vi "demo.vi"() -> ()   [LabVIEW 2019]
uses:
  <vilib>/Platform/storage/lvStorage.llb/_openFunction.ctl
  <vilib>/Platform/storage/lvStorage.llb/_openStorageWithRootAutoDetect.vi
  <vilib>/Platform/storage/lvStorage.llb/xStorage/xStorageSupp/ErrorOut.vi
  <vilib>/Platform/storage/lvStorage.llb/_queryPropPoly.vi
  <vilib>/Platform/storage/lvStorage.llb/_queryPropString.vi
  <vilib>/Platform/storage/lvStorage.llb/_queryGenericObjects.vi
  <vilib>/Platform/storage/lvStorage.llb/_loadAllDouble.vi
  <vilib>/Platform/storage/lvStorage.llb/_loadAllDdt.vi
  <vilib>/Platform/storage/Storage.llb/Get Object Info.vi
  <vilib>/Platform/storage/Storage.llb/__closeStorageFromObject.vi
  <vilib>/Instr/_visa.llb/VISA Configure Serial Port (Instr).vi
  <vilib>/Utility/file.llb/Write Delimited Spreadsheet (I64).vi
  <vilib>/Platform/storage/lvStorage.llb/xStorage/Open Data Storage/Open Data Storage.xnode
  <vilib>/Platform/storage/lvStorage.llb/xStorage/Read Data/Read Data.xnode
  <vilib>/Platform/storage/lvStorage.llb/xStorage/Close Data Storage/Close Data Storage.xnode
  phlib64.dll
panel:
  in  "If NLOS":bool
  out "Numeric":dbl
  out "String":string
  out "Index":dbl
  out "Histogram":u32[](graph)
  out "DLL Version (must be 3.0)":string caption="DLL Version"
  out "Calibration Status":string
  out "Initialization Status":string
  # "1: NLOS\n0: LOS"
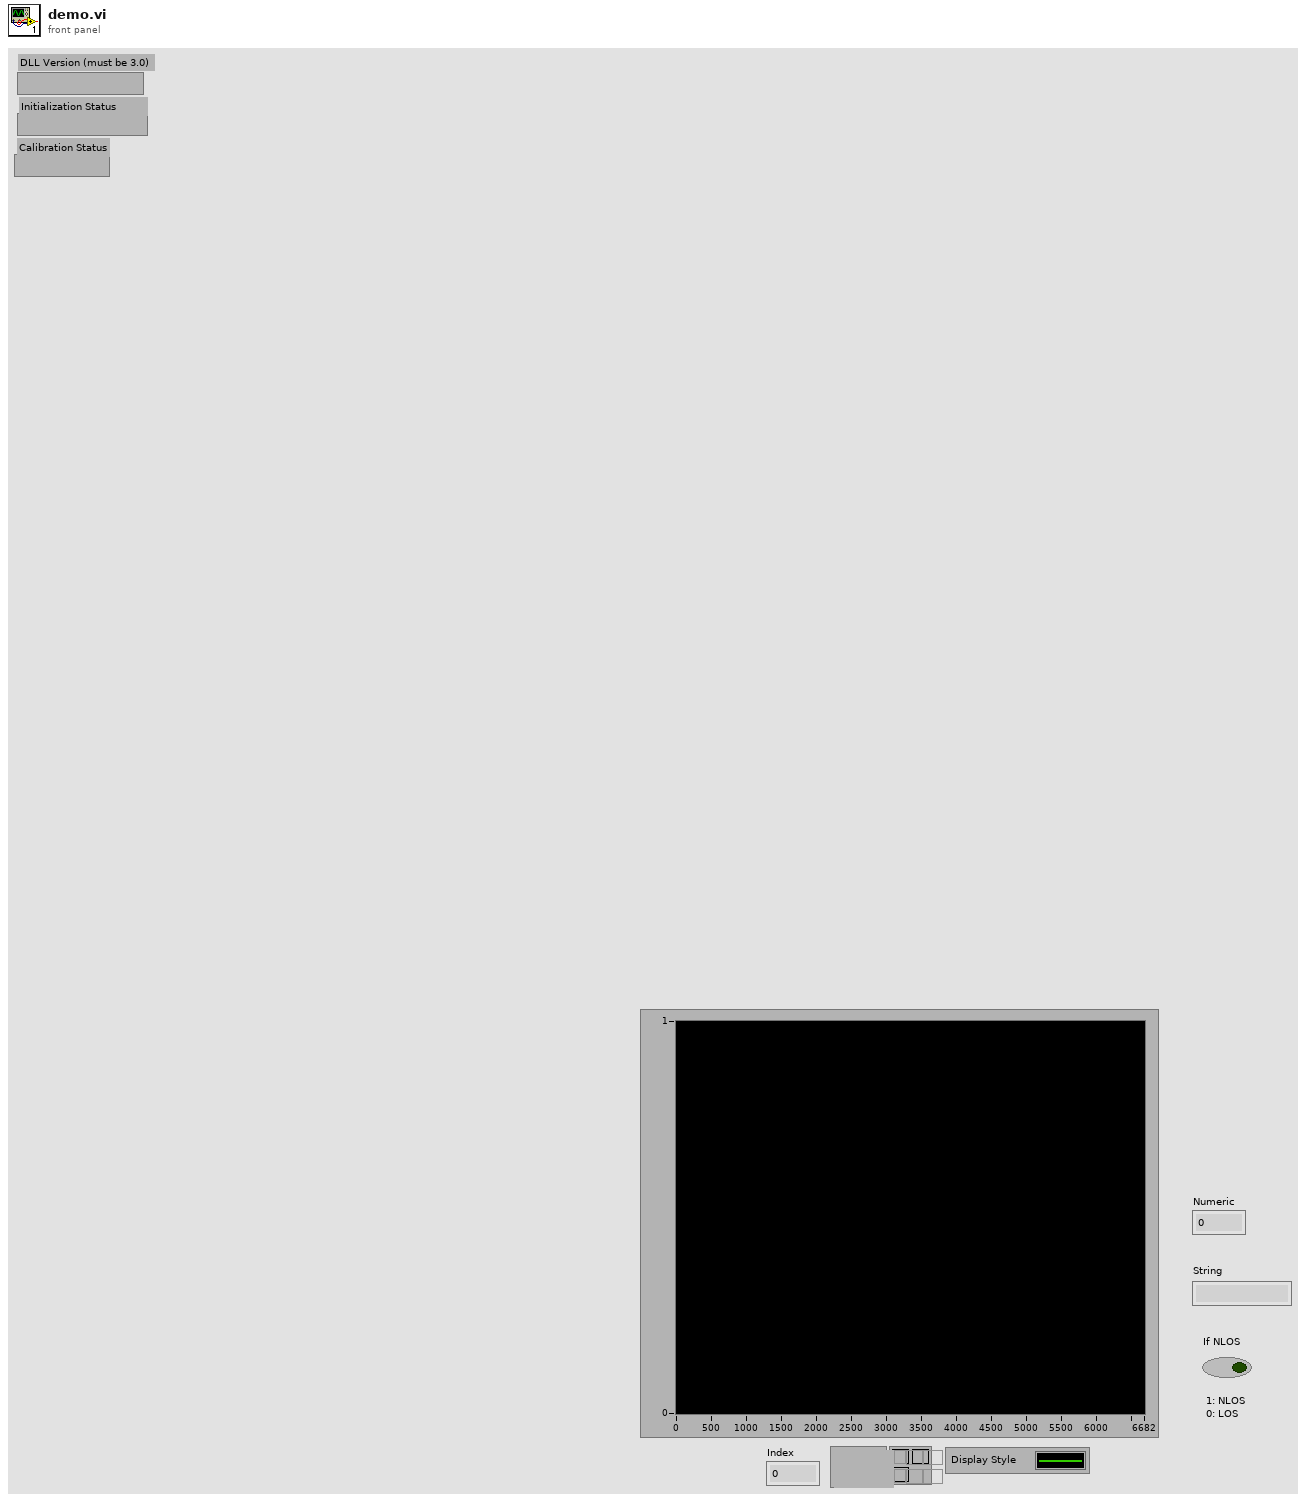
[diagram p1: front panel]
types:
  T1 = enum16{"UPDATE", "READ", "QUERY", "CREATE CHILD", "CREATE", "CONNECT", "DISCONNECT"}
  T2 = typedef "_openFunction.ctl" = enum16{"open", "open or create", "create or replace", "create", "open (read only)"}
  T3 = enum16{"open", "replace", "create", "open or create", "replace or create", "replace or create with confirmation"}
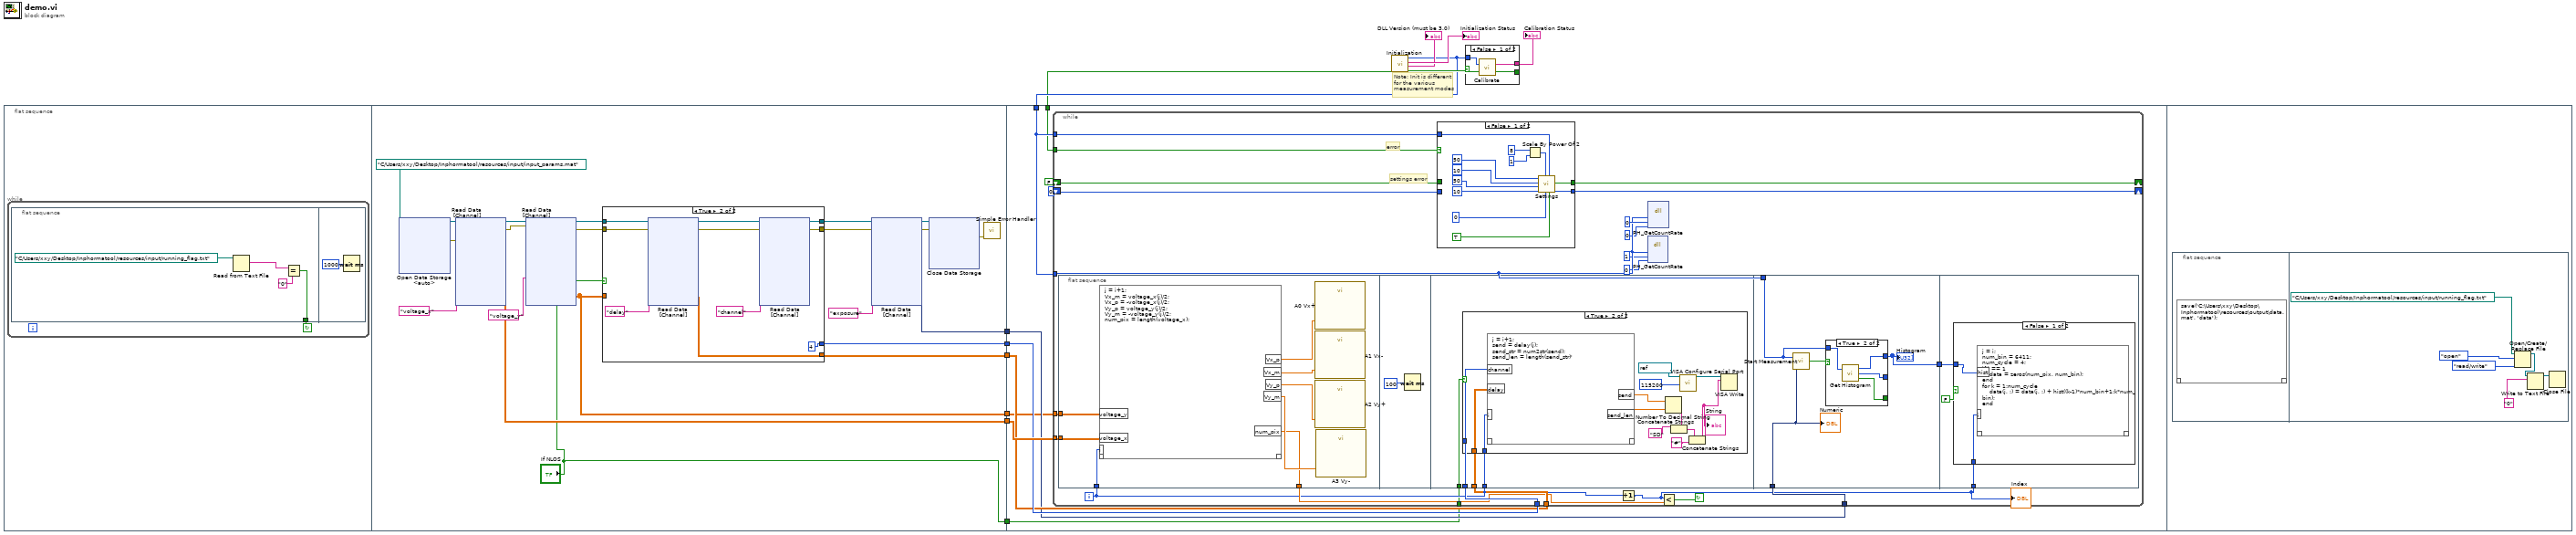
[diagram p0: block diagram]
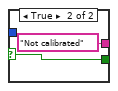
[diagram p2: hidden frame]
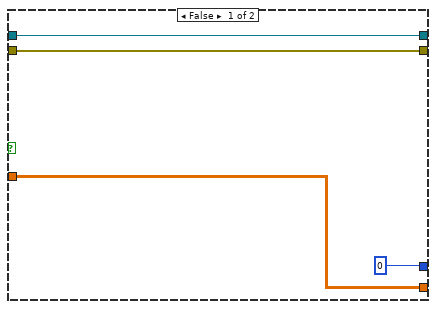
[diagram p3: hidden frame]
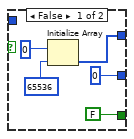
[diagram p5: hidden frame]
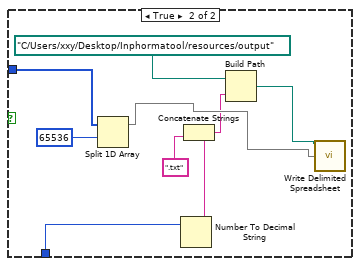
[diagram p6: hidden frame]
diagram:
  # "Note: Init is different \nfor the various\nmeasurement modes"
  n1 = flat-sequence {
    tunnel: [w36] -> w12
    tunnel: [w35] -> w11
    tunnel: [w34] -> w10
    tunnel: [w30] -> w9
    tunnel: [w21] -> w2
    tunnel: ["If NLOS"] -> w1
    tunnel: w4 -> [w171]
    tunnel: w3 -> [w170]
    tunnel: w9 -> [w164]
    tunnel: w10 -> [w166]
    tunnel: w11 -> [w165]
    tunnel: w12 -> [w167]
    tunnel: w2 -> [w163]
    tunnel: w1 -> [w162]
    frame #0 {
      n2 = while {
        stop <- w13 continue-if-true
        n3 = flat-sequence {
          tunnel: [w15] -> w13
          frame #0 {
            n4 = Read from Text File(file (use dialog)=path "C:/Users/xxy/Desktop/Inphormatool/resources/input/running_flag.txt") -> (text=w14:string)  [unwired: 3 in, 3 out]
            n5 = Equal?(x=w14, y="0") -> (x = y?=w15:bool)
          }
          frame #1 {
            n6 = Wait (ms)(milliseconds to wait=1000) -> ()  [unwired: 1 out]
          }
        }
      }
    }
    frame #1 {
      n7 = xnode "Open Data Storage\n<auto>"("file path"=path "C:/Users/xxy/Desktop/Inphormatool/resources/input/input_params.mat") -> ("storage refnum (file)"=w39:refnum<k20>, "error out"=w38:errorcluster)  [unwired: 4 in, 1 out]
      n8 = xnode "Read Data\n[Channel]"("Name"="voltage_x", "storage refnum (file)"=w39, "error in"=w38) -> ("Signal"=w36:dbl[][], "storage refnum (file) out"=w26:refnum<k20>, "error out"=w25:errorcluster)  [unwired: 3 in, 1 out]
      n9 = xnode "Read Data\n[Channel]"("Name"="voltage_y", "storage refnum (file)"=w26, "error in"=w25) -> ("Signal"=w21:dbl[][], "storage refnum (file) out"=w24:refnum<k20>, "error out"=w23:errorcluster)  [unwired: 3 in, 1 out]
      n10 = case shown="True" "If NLOS" {
        tunnel: w24 -> [w61 w71]
        tunnel: w23 -> [w60 w70]
        tunnel: [w58 w65] -> w35
        tunnel: [0 4] -> w34
        tunnel: [w61 w64] -> w32
        tunnel: [w60 w63] -> w31
        tunnel: w21 -> [w58 _]
        frame False {
        }
        frame True {
          n11 = xnode "Read Data\n[Channel]"("Name"="delay", "storage refnum (file)"=w71, "error in"=w70) -> ("Signal"=w65:dbl[][], "storage refnum (file) out"=w67:refnum<k20>, "error out"=w66:errorcluster)  [unwired: 3 in, 1 out]
          n12 = xnode "Read Data\n[Channel]"("Name"="channel", "storage refnum (file)"=w67, "error in"=w66) -> ("storage refnum (file) out"=w64:refnum<k20>, "error out"=w63:errorcluster)  [unwired: 3 in, 2 out]
        }
      }
      n13 = xnode "Read Data\n[Channel]"("Name"="exposure", "storage refnum (file)"=w32, "error in"=w31) -> ("Signal"=w30:dynamicdata, "storage refnum (file) out"=w28:refnum<k20>, "error out"=w27:errorcluster)  [unwired: 3 in, 1 out]
      n14 = xnode "Close Data Storage\n"("storage refnum (file)"=w28, "error in (no error)"=w27) -> ("error out"=w29:errorcluster)  [unwired: 1 out]
      n15 = call <vilib>:"Simple Error Handler.vi"("error in (no error)"=w29) -> ()  [unwired: 4 in, 5 out]
    }
    frame #2 {
      n16 = while {
        shift-right: [w189] -> _
        shift-left: FALSE -> [w190]
        shift-right: [w193] -> _
        shift-left: 0 -> [w192]
        tunnel: w170 -> [w191]
        tunnel: w171 -> [w188]
        tunnel: w171 -> [w186]
        tunnel: w167 -> [w182]
        tunnel: w166 -> [w181]
        tunnel: w165 -> [w178]
        tunnel: w164 -> [w180]
        tunnel: w163 -> [w177]
        tunnel: w162 -> [w172]
        i -> [w174]
        stop <- w175 continue-if-true
        # "settings error"
        # "error"
        n17 = flat-sequence {
          tunnel: w174 -> [w201]
          tunnel: w182 -> [w196]
          tunnel: w177 -> [w195]
          tunnel: [w194] -> w176
          tunnel: w181 -> [w205]
          tunnel: w178 -> [w206]
          tunnel: w174 -> [w204]
          tunnel: w172 -> [w203]
          tunnel: w186 -> [w223]
          tunnel: w180 -> [w220]
          tunnel: [w221] -> w179
          tunnel: w179 -> [w235]
          tunnel: w173 -> [w234]
          frame #0 {
            n18 = script code="j = i+1;\nVx_m = voltage_x(j)/2;\nVx_p = -voltage_x(j)/2;\nVy_p = voltage_y(j)/2;\nVy_m = -voltage_y(j)/2;\nnum_pix = length(voltage_x);"("voltage_x"=w196, "i"=w201, "voltage_y"=w195) -> ("Vx_p"=w200:dbl, "Vx_m"=w199:dbl, "Vy_p"=w198:dbl, "Vy_m"=w197:dbl, "num_pix"=w194:dbl)  [unwired: 1 in, 1 out]
            n19 = call "A0 Vx+"("data"=w200) -> ()  [unwired: 17 in, 2 out]
            n20 = call "A1 Vx-"("data"=w199) -> ()  [unwired: 17 in, 2 out]
            n21 = call "A2 Vy+"("data"=w198) -> ()  [unwired: 17 in, 2 out]
            n22 = call "A3 Vy-"("data"=w197) -> ()  [unwired: 17 in, 2 out]
          }
          frame #1 {
            n23 = Wait (ms)(milliseconds to wait=100) -> ()  [unwired: 1 out]
          }
          frame #2 {
            n24 = case shown="True" w203 {
              tunnel: w206 -> [_ w215]
              tunnel: w205 -> [_ w217]
              tunnel: w204 -> [_ w216]
              frame False {
              }
              frame True {
                n25 = script code="j = i+1;\nsend = delay(j);\nsend_str = num2str(send);\nsend_len = length(send_str)'"("channel"=w217, "delay"=w215, "i"=w216) -> ("send"=w213:dbl, "send_len"=w207:dbl)  [unwired: 1 in, 1 out]
                n26 = Number To Decimal String(number=w213, width (-)=w207) -> (decimal integer string=w211:string)
                n27 = Concatenate Strings("SD", w211) -> (w210:string)
                n28 = call-poly "VISA Configure Serial Port"("VISA resource name"=refnum<visa-resource-name> "COM8", "baud rate (9600)"=u32 115200) -> ("VISA resource name out"=w218:refnum<visa-resource-name>)  [unwired: 12 in, 1 out]
                n29 = Concatenate Strings(w210, "#") -> (w209:string)
                "String" <- w209
                n30 = VISA Write(VISA resource name=w218, write buffer=w209) -> ()  [unwired: 1 in, 3 out]
              }
            }
          }
          frame #3 {
            n31 = call "Start Measurement.vi"("Acquisition time"=w220, "DeviceIndex"=w223) -> ("DataValid"=w222:bool)
            n32 = case shown="True" w222 {
              tunnel: [w227 w232] -> w221
              tunnel: [FALSE w230] -> _
              tunnel: [u32 0 w231] -> _
              tunnel: w223 -> [_ w229]
              frame False {
                n33 = Initialize Array "Initialize Array"(u32 0, 65536) -> (w227:u32[])
              }
              frame True {
                n34 = call "Get Histogram.vi"("DeviceIndex"=w229) -> ("Histogram"=w232:u32[], "IntegralCount"=w231:i32, "Overflow"=w230:bool)  [unwired: 1 in]
              }
            }
            "Histogram" <- w221
            "Numeric" <- w220
          }
          frame #4 {
            n35 = case shown="False" FALSE {
              tunnel: w235 -> [w237 w241]
              tunnel: w234 -> [w236 w239]
              frame False {
                n36 = script code="j = i;\nnum_bin = 6411;\nnum_cycle = 4;\nif j == 1\n    data = zeros(num_pix, num_bin);\nend\nfor k = 1:num_cycle\n    data(j, :) = data(j, :) + hist((k-1)*num_bin+1:k*num_bin);\nend"("hist"=w237, "i"=w236) -> ()  [unwired: 1 in, 1 out]
              }
              frame True {
                n37 = Split 1D Array(array=w241, index=65536) -> (first subarray=w246:u32[])  [unwired: 1 out]
                n38 = Number To Decimal String(number=w239) -> (decimal integer string=w240:string)  [unwired: 1 in]
                n39 = Concatenate Strings(w240, ".txt") -> (w244:string)
                n40 = Build Path(base path=path "C:/Users/xxy/Desktop/Inphormatool/resources/output", name or relative path=w244) -> (appended path=w245:path)
                n41 = call-poly <vilib>:"Write Delimited Spreadsheet.vi"("file path (dialog if empty)"=w245, "1D data"=w246) -> ()  [unwired: 12 in, 2 out]
              }
            }
          }
        }
        n42 = case shown="False" w191 {
          tunnel: [w258 w260] -> w189
          tunnel: w190 -> [_ w260]
          tunnel: [w257 w259] -> w193
          tunnel: w192 -> [_ w259]
          tunnel: w188 -> [w254 _]
          frame False {
            n43 = Scale By Power Of 2(n=8, x=1) -> (x*2^n=w255:i32)
            n44 = call "Settings.vi"("StopOnOverflow"=TRUE, "DeviceIndex"=w254, "Range No."=0, "SyncDiv"=w255, "CFD1 zero X"=10, "CFD1 level"=50, "CFD0 zero X"=10, "CFD0 level"=50) -> ("Resolution"=w257:i32, "Error"=w258:bool)  [unwired: 2 in]
          }
          frame True {
          }
        }
        n45 = Increment(x=w174) -> (x+1=w173:i32)
        "Index" <- w173
        n46 = dll-call lib="PHLib64.dll" fn="PH_GetCountRate"("devidx"=w186, "channel"=1, "rate"=0) -> ()  [unwired: 7 in, 2 out]
        n47 = dll-call lib="PHLib64.dll" fn="PH_GetCountRate"("devidx"=w186, "channel"=0, "rate"=0) -> ()  [unwired: 7 in, 2 out]
        n48 = Less?(x=w173, y=w176) -> (x < y?=w175:bool)
      }
    }
    frame #3 {
      n49 = flat-sequence {
        frame #0 {
          n50 = script code="save('C:\\Users\\xxy\\Desktop\\Inphormatool\\resources\\output\\data.mat', 'data');"() -> ()  [unwired: 1 in, 1 out]
        }
        frame #1 {
          n51 = Open/Create/Replace File(file path (use dialog)=path "C:/Users/xxy/Desktop/Inphormatool/resources/input/running_flag.txt", operation (0:open)=T3."open", access (0:read/write)=enum16{"read/write", "read-only", "write-only"}."read/write") -> (refnum out=w264:refnum<file>)  [unwired: 3 in, 2 out]
          n52 = Write to Text File(file (use dialog)=w264, text="0") -> (refnum out=w263:refnum<file>)  [unwired: 2 in, 2 out]
          n53 = Close File(refnum=w263) -> ()  [unwired: 1 in, 2 out]
        }
      }
    }
  }
  n54 = call "Initialization.vi"() -> ("Deviceindex"=w4:i32, "Initialization Status"=→"Initialization Status":string, "DLL Version"=→"DLL Version (must be 3.0)":string, "Initialization Error"=w7:bool)  [unwired: 2 in]
  n55 = case shown="False" w7 {
    selector: w7 -> [_ w270]
    tunnel: [w269 "Not calibrated"] -> w8
    tunnel: [w268 w270] -> w3
    tunnel: w4 -> [w267 _]
    frame False {
      n56 = call "Calibrate.vi"("Deviceindex"=w267) -> ("Calib Error"=w268:bool, "Status"=w269:string)  [unwired: 1 in]
    }
    frame True {
    }
  }
  "Calibration Status" <- w8
